vi "G_DATA.vi"() -> ()   [LabVIEW 2015]
panel:
  out "path":path
  in  "load old":bool
  out "refnum_load old":refnum<k1>
  out "data_load old":T1
  in  "rate_sum":u8
  in  "rate":u8
  out "Scale.Range:Maximum":i64
  in  "save visible":bool
  in  "load visible":bool
  out "error out":errorcluster
  out "data_save":T2
  out "refnum_load":refnum<k1>
  out "refnum_save":refnum<k1>
  in  "load init":bool
  in  "saveinit":bool
  in  "size":i64=1 min=1 max=5 step=1
  in  "times":i64=1 min=1 max=5 step=1
  in  "play":bool
  out "data_load":T2
  in  "Save data":bool
  in  "Load data":bool
  in  "data pos":i64
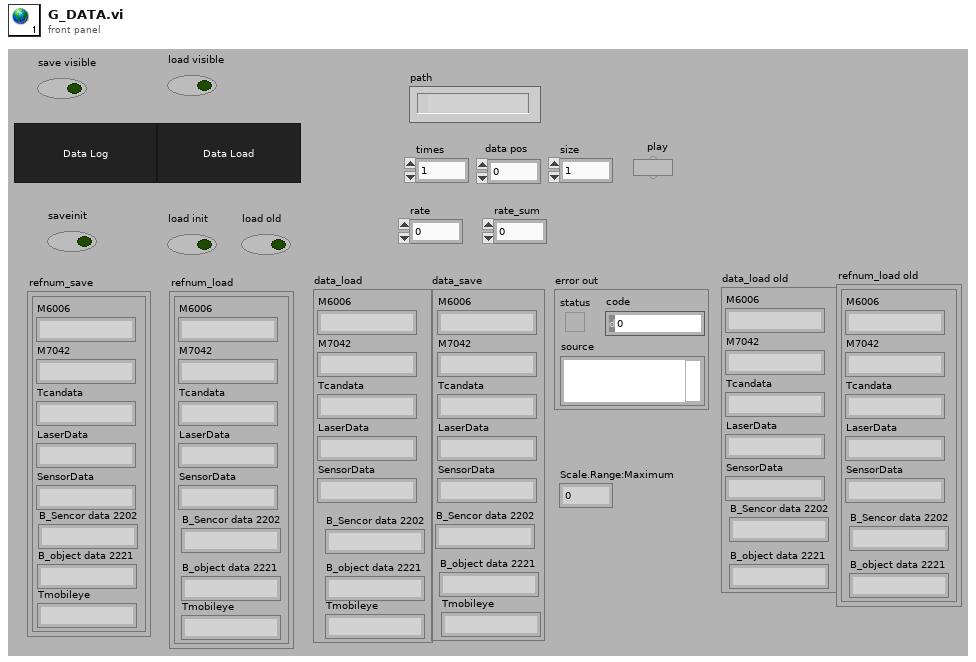
[diagram p1: front panel]
types:
  T1 = cluster{"M6006":string, "M7042":string, "Tcandata":string, "LaserData":string, "SensorData":string, "B_Sencor data 2202":string, "B_object data 2221":string}
  T2 = cluster{"M6006":string, "M7042":string, "Tcandata":string, "LaserData":string, "SensorData":string, "B_Sencor data 2202":string, "B_object data 2221":string, "Tmobileye":string}
diagram:
